vi "Close.vi"(8 "error in (no error)":errorcluster, 11 "FileStream in":refnum<class "FileStream.lvclass">) -> (0 "error out":errorcluster, 3 "FileStream out":refnum<class "FileStream.lvclass">)   [LabVIEW 2020, in "Stream.lvlib" / "FileStream.lvclass"]
uses:
  FileStream.lvclass
  FileStream.lvclass/FileStream.ctl
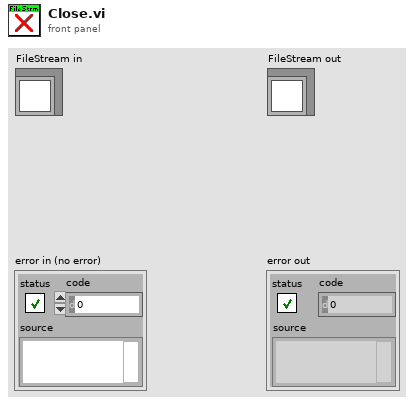
[diagram p1: front panel]
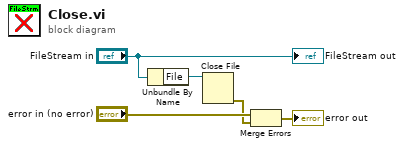
[diagram p0: block diagram]
diagram:
  n1 = Unbundle By Name("FileStream in") -> ("File"=w3:refnum<file>)
  n2 = Close File(refnum=w3) -> (error out=w1:errorcluster)  [unwired: 1 in, 1 out]
  n3 = Merge Errors("error in (no error)", w1) -> (→"error out":errorcluster)
  "FileStream out" <- "FileStream in"
